vi "main.vi"() -> ()   [LabVIEW 2024]
uses:
  stateMachineStates.ctl
  states.ctl
panel:
  in  "minus":bool
  out "Counter":i32
  in  "stop":bool
  in  "count":bool
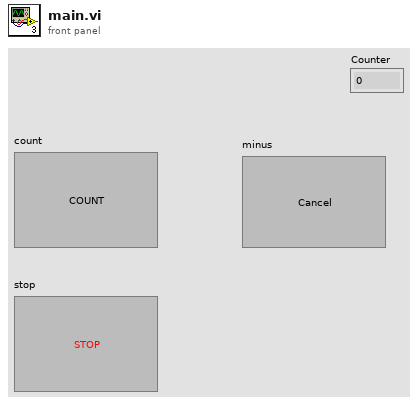
[diagram p1: front panel]
types:
  T1 = typedef "stateMachineStates.ctl" = enum16{"INIT", "IDLE", "EXIT"}
  T2 = typedef "states.ctl" = enum16{"SET", "GET", "INC", "DEC"}
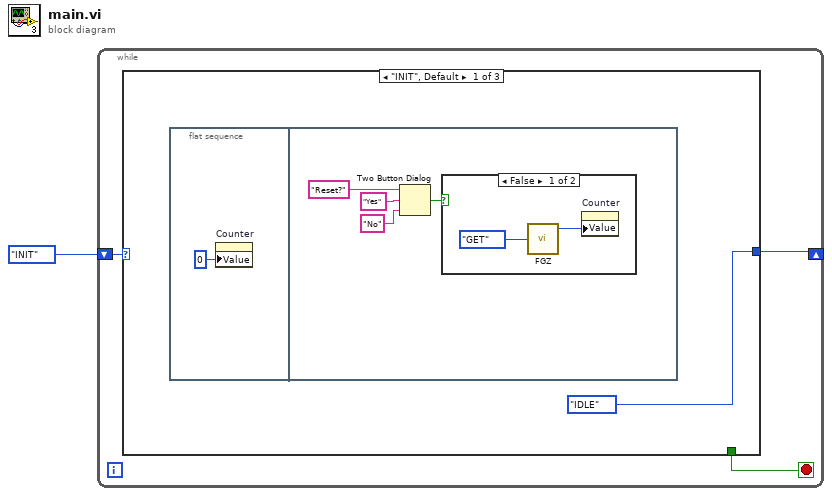
[diagram p0: block diagram]
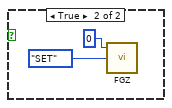
[diagram p2: hidden frame]
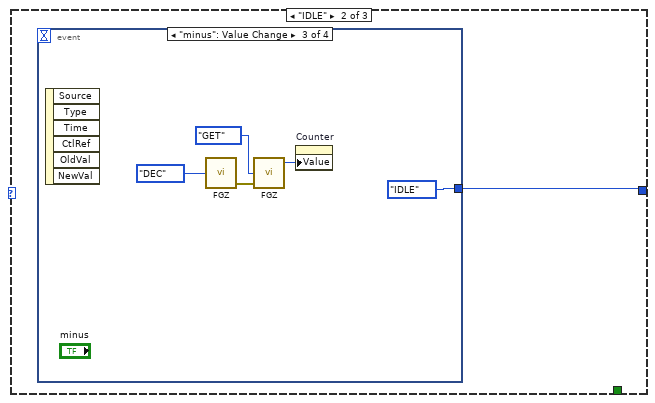
[diagram p3: hidden frame]
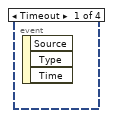
[diagram p4: hidden frame]
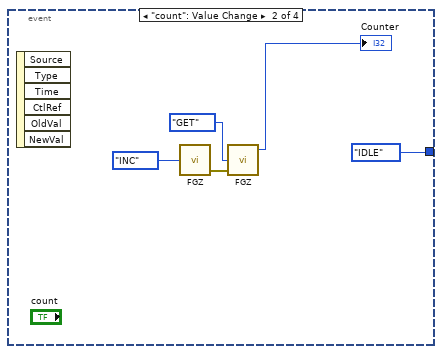
[diagram p5: hidden frame]
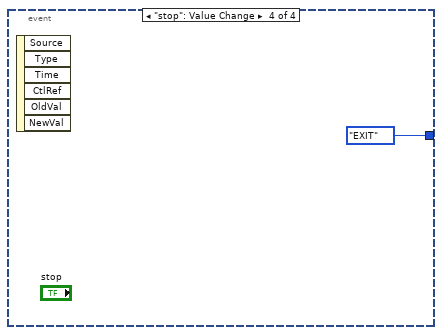
[diagram p6: hidden frame]
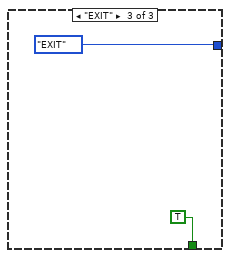
[diagram p7: hidden frame]
diagram:
  n1 = while {
    shift-right: [w3] -> _
    shift-left: stateMachineStates."INIT" -> [w4]
    stop <- w2 stop-if-true
    n2 = case shown="\"INIT\", Default" w4 {
      tunnel: [stateMachineStates."IDLE" w15 stateMachineStates."EXIT"] -> w3
      tunnel: [_ _ TRUE] -> w2
      frame "INIT", Default {
        n3 = flat-sequence {
          frame #0 {
            n4 = property on="Counter" class="DigNum (strict)"("Value"=0 ("Counter")) -> ()  [unwired: 2 in, 2 out]
          }
          frame #1 {
            n5 = Two Button Dialog(message="Reset?", 1:"No" ("F button name (\"Cancel\")"), 2:"Yes" ("T button name (\"OK\")")) -> (T button?=w10:bool)
            n6 = case shown="False" w10 {
              frame False {
                n7 = call "FGZ.vi"("state"=states."GET") -> ("Output"=w12:i32)  [unwired: 3 in, 1 out]
                n8 = property on="Counter" class="DigNum (strict)"("Value"=w12) -> ()  [unwired: 2 in, 2 out]
              }
              frame True {
                n9 = call "FGZ.vi"("state"=states."SET", "Input"=0) -> ()  [unwired: 2 in, 2 out]
              }
            }
          }
        }
      }
      frame "IDLE" {
        n10 = event shown="[2] \"minus\": Value Change" {
          selector: _ -> [_ _ _ _]
          dyn-events: _ -> [_ _ _ _]
          timeout: _ -> [_ _ _ _]
          tunnel: [_ stateMachineStates."IDLE" stateMachineStates."IDLE" stateMachineStates."EXIT"] -> w15
          event Timeout {
            n11 = event-data() -> ()  [unwired: 1 in, 3 out]
          }
          event "count": Value Change {
            n12 = event-data() -> ()  [unwired: 1 in, 6 out]
            n13 = call "FGZ.vi"("state"=states."INC") -> ("error out"=w18:errorcluster)  [unwired: 3 in, 1 out]
            n14 = call "FGZ.vi"("error in (no error)"=w18, "state"=states."GET") -> ("Output"=→"Counter":i32)  [unwired: 2 in, 1 out]
          }
          event "minus": Value Change {
            n15 = event-data() -> ()  [unwired: 1 in, 6 out]
            n16 = call "FGZ.vi"("state"=states."DEC") -> ("error out"=w25:errorcluster)  [unwired: 3 in, 1 out]
            n17 = call "FGZ.vi"("error in (no error)"=w25, "state"=states."GET") -> ("Output"=w24:i32)  [unwired: 2 in, 1 out]
            n18 = property on="Counter" class="DigNum (strict)"("Value"=w24) -> ()  [unwired: 2 in, 2 out]
          }
          event "stop": Value Change {
            n19 = event-data() -> ()  [unwired: 1 in, 6 out]
          }
        }
      }
      frame "EXIT" {
      }
    }
  }
